vi "PH_Synchrolock_Watch.evt call Set Limit.vi"(0 "i ref in":refnum<vi>, 2 "Instance":string="N/A", 3 "Limit to set":T1 items=["Mean Phase upper Limit", "Mean Phase lower Limit", "RF Amplutude lower Limit", "Mira Amplidute upper Limit", "Mira Amplidute lower Limit"], 4 "Limit":dbl, 5 "error in (no error)":errorcluster) -> (14 "i ref out":refnum<vi>, 19 "error out":errorcluster)   [LabVIEW 2014, in "PH_Synchrolock_Watch.lvlib"]
doc: "This VI sets the instance remotely controlled by a simple call."
uses:
  PH_Synchrolock_Watch.Limit to set.ctl
  CS_Core/CSSystem/CoreLib/CoreLib.double 2 byte array.vi
  CS_Core/CSSystem/CoreLib/CoreLib.short 2 byte array.vi
  PH_Synchrolock_Watch.lvlib
  CS_Core/CSSystem/CoreLib/CoreLib.lvlib
  CS_Core/BaseProcess/BaseProcess.lvlib
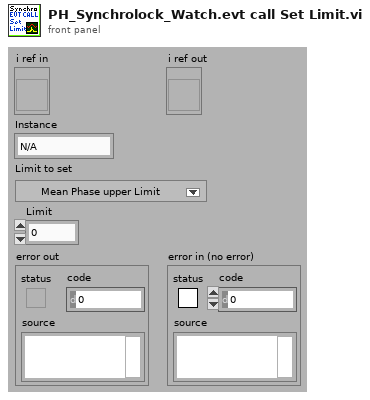
[diagram p1: front panel]
types:
  T1 = typedef "PH_Synchrolock_Watch.lvlib/PH_Synchrolock_Watch.Limit to set.ctl" = i16
  T2 = typedef "CoreDefs.rawDataType.ctl" = i8[]
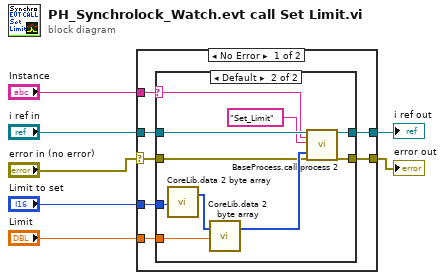
[diagram p0: block diagram]
diagram:
  n1 = case shown="No Error" "error in (no error)" {
    selector: "error in (no error)" -> [w11 w28]
    tunnel: [w14 w27] -> w7
    tunnel: [w13 w28] -> w6
    tunnel: "i ref in" -> [w12 w27]
    tunnel: "Instance" -> [w10 _]
    tunnel: "Limit" -> [w9 _]
    tunnel: "Limit to set" -> [w8 _]
    frame No Error {
      n2 = case shown="Default" w10 {
        selector: w10 -> [_ w20]
        tunnel: [w16 w26] -> w14
        tunnel: [w15 w25] -> w13
        tunnel: w12 -> [w16 w24]
        tunnel: w11 -> [w15 w21]
        tunnel: w9 -> [_ w19]
        tunnel: w8 -> [_ w18]
        frame "N/A" {
        }
        frame Default {
          n3 = call-poly "CoreLib.data 2 byte array.vi"("i16"=w18) -> ("byteArray out"=w17:T2)  [unwired: 18 in]
          n4 = call-poly "CoreLib.data 2 byte array.vi"("byteArray"=w17, "f64"=w19) -> ("byteArray out"=w22:T2)  [unwired: 17 in]
          n5 = call "BaseProcess.call process 2.vi"("i ref in"=w24, "Object"=w20, "Selector"="Set_Limit", "Data"=w22, "error in (no error)"=w21) -> ("i ref out"=w26:refnum<vi>, "error out"=w25:errorcluster)  [unwired: 13 in]
        }
      }
    }
    frame Error {
    }
  }
  "error out" <- w6
  "i ref out" <- w7
